vi "rwfm_AcqConfig(Ss).vi"(5 "Samples per Channel":i32=1000, 7 "Sample Mode":enum16{"Finite Samples", "Continuous Samples"}(ring), 8 "error in":errorcluster, 9 "Sample Rate S/s":u32, 10 "Sampling Info In":T2, 11 "Dynamic FPGA Ref":T1) -> (0 "error out":errorcluster, 2 "Sampling Info Out":T2, 3 "Dynamic FPGA Ref Out":T1, 4 "Sample Rate (u32)":u32)   [LabVIEW 2017, in "cRIOWfmLib.lvlib"]
doc: "This VI sets the sampling mode (either finite or continuous) and transfers sampling rate to the FPGA. Pay close attention to the polymorphic instance used by this VI. Some NI C Series modules support sample rates that are integer divisions of 51.2 kS/s and some support sample rates that are integer divisions of 50 kS/s. When you synchronize multiple Delta Sigma modules together, the supported rates of all modules are equal to the supported rates of the master. Timebase sharing is configured through the LabVIEW project.\n\nIf the overall data rate is not dictated by a Delta Sigma-based C Series module, be sure to select the \"Non Delta Sigma\" instance of this VI."
uses:
  <vilib>/addons/InsightCM/Devices/Shared/Cms/cRIOWfmAcq/cRIOWfmLib.lvlib
  <vilib>/addons/InsightCM/Devices/Shared/Cms/cRIOWfmAcq/subVIs/RIO Wfm Cust Ctrls/rwfm_SamplingInfo.ctl
  <vilib>/addons/InsightCM/Devices/Shared/Cms/cRIOWfmAcq/subVIs/RIO Wfm Cust Ctrls/rwfm_DynamicFPGAref2.ctl
  <vilib>/Utility/error.llb/Error Cluster From Error Code.vi
  <vilib>/rvi/errors/niLvFpgaAdjustHostInterfaceError.vi
  <vilib>/rvi/interface/nirviReadWriteControl/nirviReadWriteControl.xnode
  NiFpgaLv.dll
  <vilib>/rvi/interface/Simulation/niFpgaSimulationCallBeginRW.vi
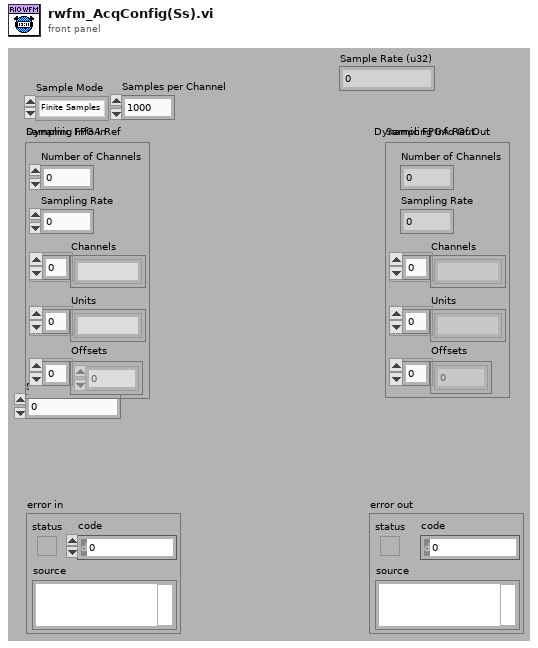
[diagram p1: front panel]
types:
  T1 = typedef "cRIOWfmLib.lvlib/rwfm_DynamicFPGAref2.ctl" = refnum<k20>
  T2 = typedef "cRIOWfmLib.lvlib/rwfm_SamplingInfo.ctl" = cluster{"Number of Channels":i32, "Sampling Rate":dbl, "Channels":string[], "Units":string[], "Offsets":sgl[]}
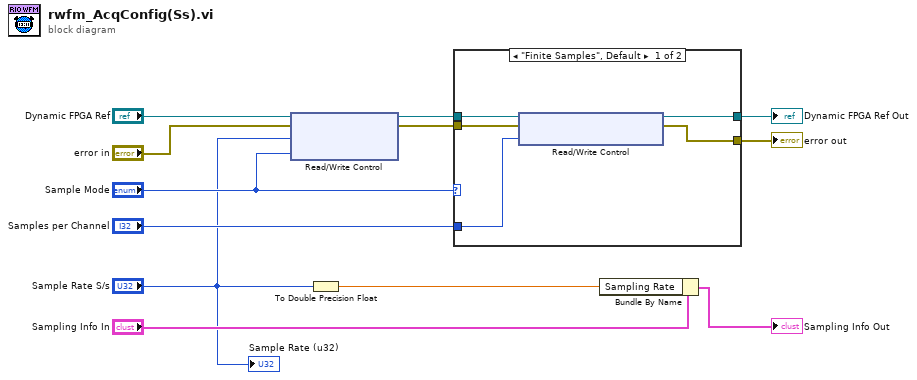
[diagram p0: block diagram]
diagram:
  n1 = xnode "Read/Write Control"("FPGA VI Reference In"="Dynamic FPGA Ref", "error in"="error in", "Data Rate [S/s]"="Sample Rate S/s", "Acquisition Type"="Sample Mode") -> ("FPGA VI Reference Out"=w12:T1, "error out"=w11:errorcluster)
  n2 = To Double Precision Float(number="Sample Rate S/s") -> (double precision float=w3:dbl)
  n3 = case shown="\"Finite Samples\", Default" "Sample Mode" {
    tunnel: w12 -> [w17 w19]
    tunnel: w11 -> [w16 w18]
    tunnel: [w13 w19] -> w4
    tunnel: [w15 w18] -> w8
    tunnel: "Samples per Channel" -> [w14 _]
    frame "Finite Samples", Default {
      n4 = xnode "Read/Write Control"("FPGA VI Reference In"=w17, "error in"=w16, "Samps per Chan [Finite]"=w14) -> ("FPGA VI Reference Out"=w13:T1, "error out"=w15:errorcluster)
    }
    frame "Continuous Samples" {
    }
  }
  "error out" <- w8
  "Dynamic FPGA Ref Out" <- w4
  n5 = Bundle By Name(cluster="Sampling Info In", "Sampling Rate"=w3) -> (→"Sampling Info Out":T2)
  "Sample Rate (u32)" <- "Sample Rate S/s"
